vi "Execute.vi"(8 "error in (no error)":errorcluster, 10 ".NET:ContactAndRegisterWithNmaSapService.SerialNoRegisterRequest":T1, 11 "ContactAndRegisterWithNmaSapService refnum":refnum<k24>) -> (0 "error out":errorcluster, 2 ".NET:ContactAndRegisterWithNmaSapService.SerialNoRegisterResponse":T2, 3 "ContactAndRegisterWithNmaSapService refnum out":refnum<k24>)   [LabVIEW 2023, in "ContactAndRegisterWithNmaSapService.lvlib"]
uses:
  <userlib>/WebService/_ContactAndRegisterWithNmaSapService/ContactAndRegisterWithNmaSapService.lvlib
  <userlib>/WebService/_ContactAndRegisterWithNmaSapService/ContactAndRegisterWithNmaSapService.dll
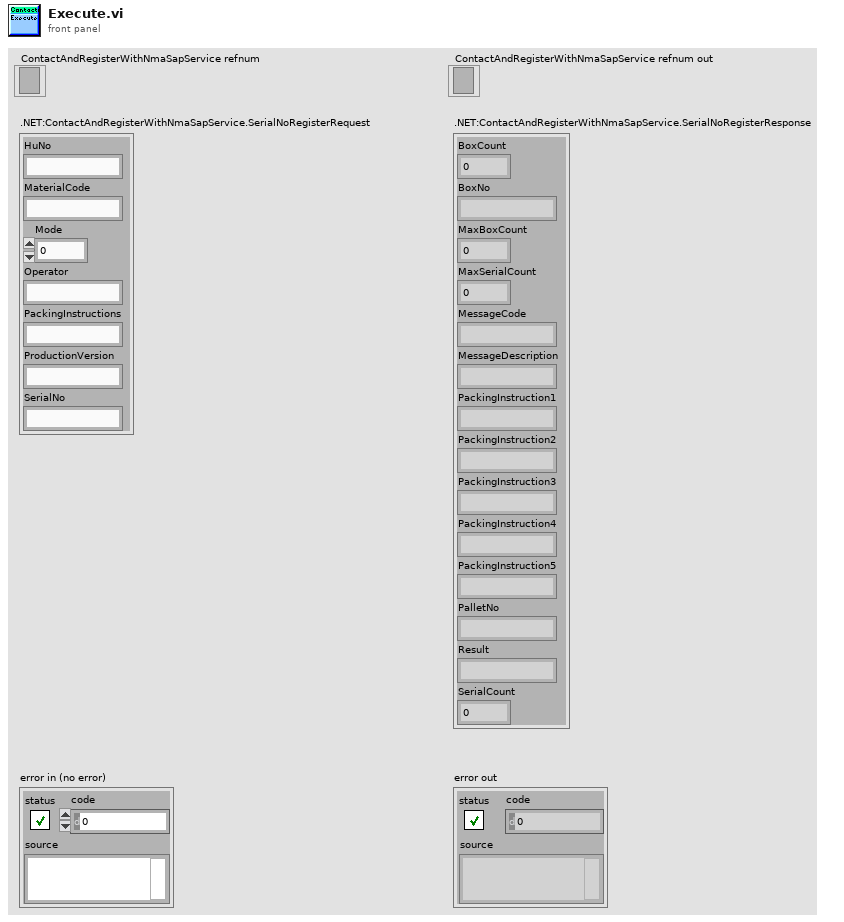
[diagram p1: front panel]
types:
  T1 = cluster{"HuNo":string, "MaterialCode":string, "Mode":i32, "Operator":string, "PackingInstructions":string, "ProductionVersion":string, "SerialNo":string}
  T2 = cluster{"BoxCount":i32, "BoxNo":string, "MaxBoxCount":i32, "MaxSerialCount":i32, "MessageCode":string, "MessageDescription":string, "PackingInstruction1":string, "PackingInstruction2":string, "PackingInstruction3":string, "PackingInstruction4":string, "PackingInstruction5":string, "PalletNo":string, "Result":string, "SerialCount":i32}
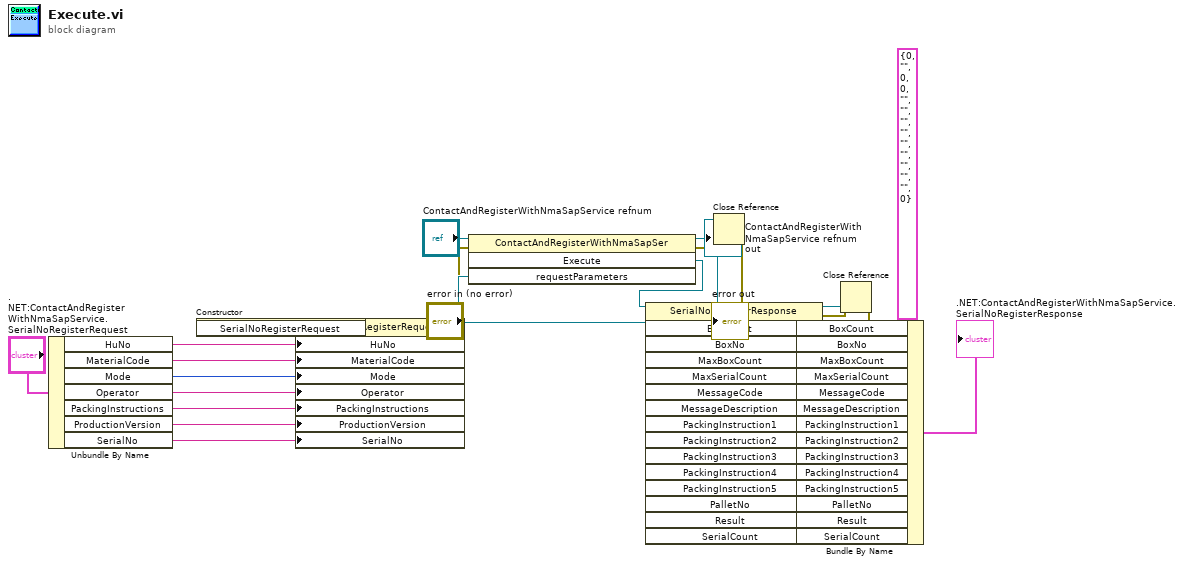
[diagram p0: block diagram]
diagram:
  n1 = Unbundle By Name(".NET:ContactAndRegisterWithNmaSapService.SerialNoRegisterRequest") -> ("HuNo"=w14:string, "MaterialCode"=w13:string, "Mode"=w12:i32, "Operator"=w11:string, "PackingInstructions"=w10:string, "ProductionVersion"=w9:string, "SerialNo"=w8:string)
  n2 = constructor class="SerialNoRegisterRequest"(error in="error in (no error)") -> (reference out=w18:refnum<k24>, error out=w17:errorcluster)  [unwired: 2 in, 1 out]
  n3 = property class="SerialNoRegisterRequest"(reference=w18, error in=w17, "HuNo"=w14, "MaterialCode"=w13, "Mode"=w12, "Operator"=w11, "PackingInstructions"=w10, "ProductionVersion"=w9, "SerialNo"=w8) -> (reference out=w16:refnum<k24>, error out=w6:errorcluster)
  n4 = invoke class="ContactAndRegisterWithNmaSapSer" method="Execute"(reference="ContactAndRegisterWithNmaSapService refnum", error in=w6, "requestParameters"=w16) -> (reference out=→"ContactAndRegisterWithNmaSapService refnum out":refnum<k24>, error out=w5:errorcluster, "Execute"=w35:refnum<k24>)  [unwired: 1 in, 1 out]
  n5 = Close Reference(reference=w16, error in (no error)=w5) -> (error out=w4:errorcluster)
  n6 = property class="SerialNoRegisterResponse"(reference=w35, error in=w4) -> (reference out=w3:refnum<k24>, error out=w2:errorcluster, "BoxCount"=w32:i32, "BoxNo"=w31:string, "MaxBoxCount"=w30:i32, "MaxSerialCount"=w29:i32, "MessageCode"=w28:string, "MessageDescription"=w27:string, "PackingInstruction1"=w26:string, "PackingInstruction2"=w25:string, "PackingInstruction3"=w24:string, "PackingInstruction4"=w23:string, "PackingInstruction5"=w22:string, "PalletNo"=w21:string, "Result"=w20:string, "SerialCount"=w19:i32)
  n7 = Bundle By Name(cluster=T2 {"BoxCount"=0, "BoxNo"="", "MaxBoxCount"=0, "MaxSerialCount"=0, "MessageCode"="", "MessageDescription"="", "PackingInstruction1"="", "PackingInstruction2"="", "PackingInstruction3"="", "PackingInstruction4"="", "PackingInstruction5"="", "PalletNo"="", "Result"="", "SerialCount"=0} (".NET:ContactAndRegisterWithNmaSapService.SerialNoRegisterResponse"), "BoxCount"=w32, "BoxNo"=w31, "MaxBoxCount"=w30, "MaxSerialCount"=w29, "MessageCode"=w28, "MessageDescription"=w27, "PackingInstruction1"=w26, "PackingInstruction2"=w25, "PackingInstruction3"=w24, "PackingInstruction4"=w23, "PackingInstruction5"=w22, "PalletNo"=w21, "Result"=w20, "SerialCount"=w19) -> (→".NET:ContactAndRegisterWithNmaSapService.SerialNoRegisterResponse":T2)
  n8 = Close Reference(reference=w3, error in (no error)=w2) -> (error out=→"error out":errorcluster)
